vi "VCS Set Object.vi"(0 "axis In":cluster{"keyHandle":u32, "nodeId":u16}={"keyHandle"=0, "nodeId"=1}, 5 "object in":T1 {"object subIndex" format="%x"; "object index" format="%x"}, 11 "error in (no error)":errorcluster) -> (4 "axis Out":cluster{"keyHandle":u32, "nodeId":u16}={"keyHandle"=0, "nodeId"=1}, 15 "error out":errorcluster)   [LabVIEW 2019, in "maxonEPOS.lvlib"]
doc: "<B>VCS Set Object</B> writes an object value at the given index and sub index from object dictionary."
uses:
  Examples/maxonEPOS.lvlib
  Resources/EposCmd64.dll
  Resources/EposCmd.dll
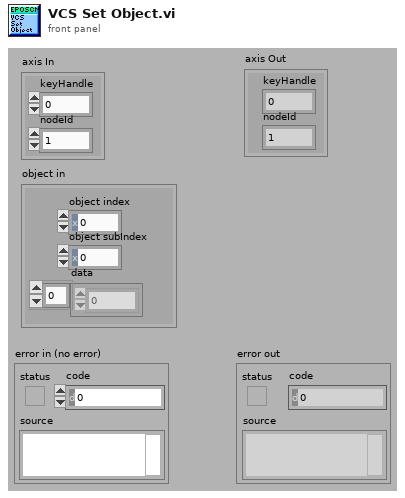
[diagram p1: front panel]
types:
  T1 = cluster{"object index":u16, "object subIndex":u8, "data":u8[]}
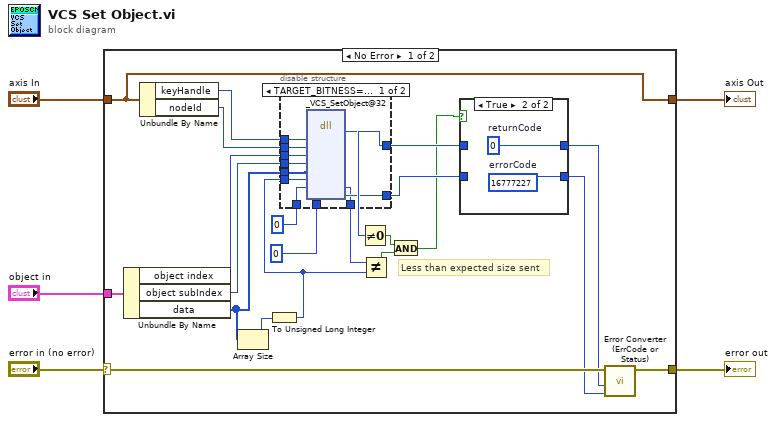
[diagram p0: block diagram]
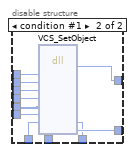
[diagram p2: hidden frame]
diagram:
  n1 = case shown="No Error" "error in (no error)" {
    selector: "error in (no error)" -> [w26 w54]
    tunnel: [w25 w54] -> w4
    tunnel: "axis In" -> [w11 w53]
    tunnel: "object in" -> [w24 _]
    tunnel: [w11 w53] -> w1
    frame No Error {
      # "Less than expected size sent"
      n2 = Unbundle By Name(w24) -> ("object index"=w21:u16, "object subIndex"=w20:u8, "data"=w19:u8[])
      n3 = Unbundle By Name(w11) -> ("keyHandle"=w23:u32, "nodeId"=w22:u16)
      n4 = Array Size(array=w19) -> (size(s)=w7:i32)
      n5 = To Unsigned Long Integer(number=w7) -> (unsigned 32bit integer=w6:u32)
      n6 = disable-structure shown="TARGET_BITNESS==32, Standard" {
        disable-tunnel: w23 -> [w37 w48]
        disable-tunnel: w22 -> [w36 w47]
        disable-tunnel: w21 -> [w35 w46]
        disable-tunnel: w20 -> [w34 w45]
        disable-tunnel: w19 -> [w33 w44]
        disable-tunnel: [w32 w43] -> w18
        disable-tunnel: [w31 w42] -> w16
        disable-tunnel: [w30 w41] -> w15
        disable-tunnel: u32 0 ("pNbOfBytesWritten") -> [w29 w40]
        disable-tunnel: u32 0 ("pErrorCode") -> [w28 w39]
        disable-tunnel: w6 -> [w27 w38]
        frame condition #0 (active) {
          n7 = dll-call lib="C:/workspace/project/scancon/sw/SSI_Tool/InstrumentsInterfaces/Motordriver/maxon EPOS/Resources/EposCmd.dll" fn="_VCS_SetObject@32"("KeyHandle"=w37, "NodeId"=w36, "ObjectIndex"=w35, "ObjectSubIndex"=w34, "Data"=w33, "NbOfBytesToWrite"=w27, "pNbOfBytesWritten"=w29, "pErrorCode"=w28) -> ("Rückgabetyp"=w30:i32, "pNbOfBytesWritten"=w31:u32, "pErrorCode"=w32:u32)  [unwired: 9 in, 2 out]
        }
        frame condition #1 {
          n8 = dll-call lib="C:/Temp/Tests/LabVIEW/maxon EPOS/Resources/EposCmd64.dll" fn="VCS_SetObject" ("EposCmd.dll:_VCS_SetObject@32")("KeyHandle"=w48, "NodeId"=w47, "ObjectIndex"=w46, "ObjectSubIndex"=w45, "Data"=w44, "NbOfBytesToWrite"=w38, "pNbOfBytesWritten"=w40, "pErrorCode"=w39) -> ("Rückgabetyp"=w41:i32, "pNbOfBytesWritten"=w42:u32, "pErrorCode"=w43:u32)  [unwired: 9 in, 2 out]
        }
      }
      n9 = Not Equal To 0?(x=w15) -> (x != 0?=w13:bool)
      n10 = Not Equal?(x=w16, y=w6) -> (x != y?=w14:bool)
      n11 = And(x=w13, y=w14) -> (x .and. y?=w12:bool)
      n12 = case shown="True" w12 {
        tunnel: [w50 w52] -> w8
        tunnel: [w49 w51] -> w17
        tunnel: w15 -> [w50 _]
        tunnel: w18 -> [w49 _]
        frame False {
        }
        frame True {
          w51 = u32 16777227  # errorCode
          w52 = 0  # returnCode
        }
      }
      n13 = call "Error Converter (ErrCode or Status).vi"("error code"=w17, "return type"=w8, "error in (no error)"=w26) -> ("error out"=w25:errorcluster)  [unwired: 7 in]
    }
    frame Error {
    }
  }
  "error out" <- w4
  "axis Out" <- w1
